vi "Rotate Points.vi"() -> ()   [LabVIEW 2020]
uses:
  Vec3.ctl
  <vilib>/Analysis/Matrix/Numeric/Conversions/Array To Matrix - RA.vi
  <vilib>/Analysis/Matrix/Numeric/Multiply/Multiply - RM,RM.vi
  <vilib>/Analysis/Matrix/Numeric/Conversions/Matrix To Array - RM.vi
  <vilib>/Analysis/Matrix/NI_Matrix.lvlib
panel:
  in  "Rotation":T1
  out "Rotated":T1[](array[typedef])
  in  "Points":T1[](array[typedef])
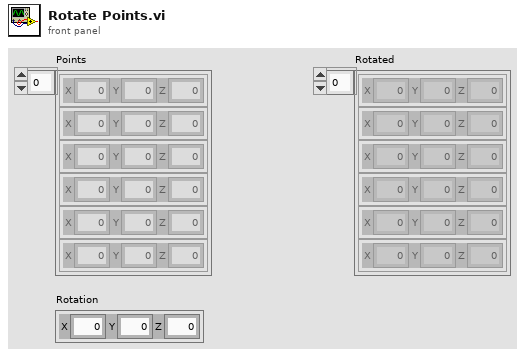
[diagram p1: front panel]
types:
  T1 = typedef "Vec3.ctl" = cluster{"X":dbl, "Y":dbl, "Z":dbl}
  T2 = typedef "NI_Matrix.lvlib/RealMatrix.ctl" = dbl[][]
  T3 = cluster{"Real 2D Array[0]":dbl, "Real 2D Array[1]":dbl, "Real 2D Array[2]":dbl}
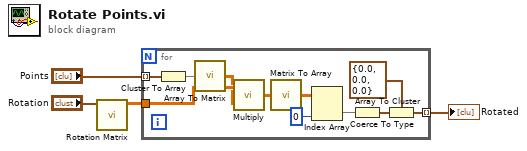
[diagram p0: block diagram]
diagram:
  n1 = call "Rotation Matrix.vi"("Rotation"="Rotation") -> ("X*Y*Z"=w2:T2)  [unwired: 10 in]
  n2 = for {
    tunnel: "Points" -> [w15] mode=indexing
    tunnel: w2 -> [w13]
    tunnel: [w5] -> w1 mode=indexing
    n3 = Cluster To Array(cluster=w15) -> (array=w14:dbl[])
    n4 = call-poly <vilib>:"Array To Matrix.vi"("Real 1D Array"=w14) -> ("Real Matrix (Column Vector)"=w12:T2)
    n5 = call-poly <vilib>:"Multiply.vi"("Real Matrix B"=w12, "Real Matrix A"=w13) -> ("A * B"=w11:T2)
    n6 = call-poly <vilib>:"Matrix To Array.vi"("Real Matrix"=w11) -> ("Real 2D Array"=w10:dbl[][])
    n7 = Index Array(array=w10, index (col)=0 ("disabled index (col)")) -> (element=w8:dbl[])  [unwired: 1 in]
    n8 = Array To Cluster(array=w8) -> (cluster=w7:T3)
    n9 = Coerce To Type(0:w7, 1:T1 {"X"=0.0, "Y"=0.0, "Z"=0.0} ("Position")) -> (2:w5:T1)
  }
  "Rotated" <- w1
